vi "Pre Launch Init.vi"(11 "LoggingActor in":refnum<class "LoggingActor.lvclass">) -> (0 "error out":errorcluster, 3 "LoggingActor out":refnum<class "LoggingActor.lvclass">)   [LabVIEW 2022 SP3, in "LoggingActor.lvlib" / "LoggingActor.lvclass"]
doc: "(<B>Filename</B>: Actor Framework.lvlib:Actor.lvclass:Pre Launch Init.vi)\n\nDefines behavior that occurs after the Launch Actor method is invoked but before the actor's Actor Core method begins running.\n\nThe Pre Launch Init method is guaranteed to finish before the Launch Actor method returns to its caller and before the actor itself receives any messages. Any references that the Pre Launch Init method obtains are guaranteed to have the same lifetime as the actor itself. Any errors that the Pre Launch Init method returns will abort the launch.\n\nBy default, this method does nothing. A descendant class may override it to define behavior."
uses:
  LoggingActor.lvclass
  Logger/Source/Logger/_Level.ctl
  LoggingActor.lvclass/LoggingActor.ctl
  Logger/Source/FileHandler/FileHandler.lvclass
  C:/Users/jakub/repos/gh/sw4sys/lv-logging-actor/Logger/Source/Handler/Handler.lvclass
  <vilib>/ActorFramework/Actor/Actor.lvclass
  Logger/Source/Logger/Logger.lvclass
  DateTime/Source/DateTime.lvlib
  Logger/Source/Handler/Handler.lvclass
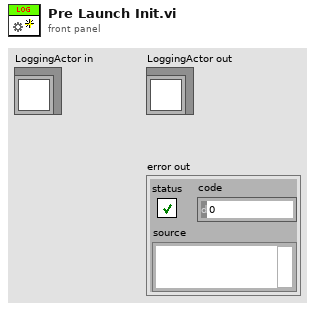
[diagram p1: front panel]
types:
  T1 = typedef "Logger.lvlib/Logger.lvclass/_Level.ctl" = enum16{"NOTSET", "DEBUG", "INFO", "WARNING", "ERROR", "CRITICAL"}
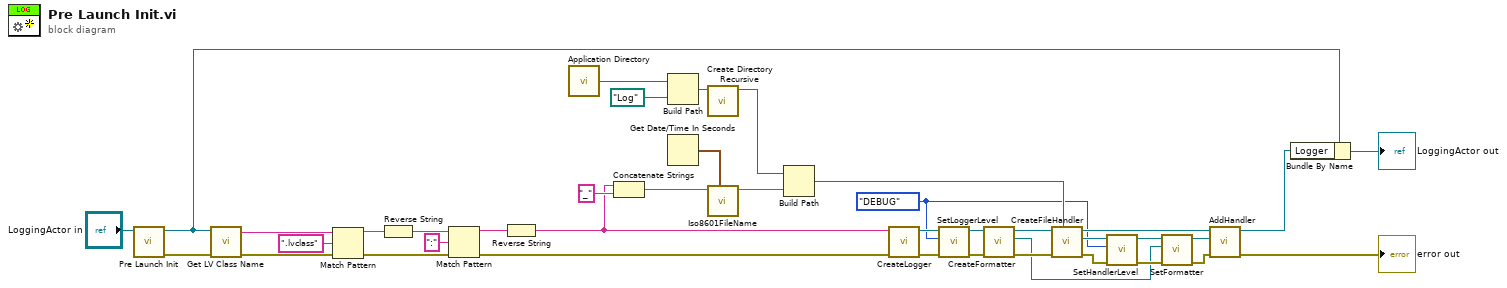
[diagram p0: block diagram]
diagram:
  w8 = _Level."DEBUG" ("Level")
  n1 = call-parent "Pre Launch Init.vi"("Actor in"="LoggingActor in") -> ("error out"=w36:errorcluster, "Actor out"=w10:refnum<class "LoggingActor.lvclass">)  [unwired: 9 in]
  n2 = call <vilib>:"Get LV Class Name.vi"("error in (no error)"=w36, "object"=w10) -> ("error out"=w35:errorcluster, "class name"=w4:string)  [unwired: 8 in]
  n3 = Match Pattern(string=w4, regular expression=".lvclass") -> (before substring=w6:string)  [unwired: 1 in, 3 out]
  n4 = Reverse String(1:w6) -> (0:w3:string)
  n5 = Match Pattern(string=w3, regular expression=":") -> (before substring=w2:string)  [unwired: 1 in, 3 out]
  n6 = Reverse String(1:w2) -> (0:w1:string)
  n7 = call <vilib>:"Application Directory.vi"() -> ("Application Directory"=w32:path)
  n8 = Concatenate Strings(w1, "_" ("Prefix ('')")) -> (w25:string)
  n9 = Build Path(base path=w32, name or relative path=path "Log") -> (appended path=w30:path)
  n10 = Get Date/Time In Seconds() -> (seconds since 1Jan1904=w28:timestamp)
  n11 = call <vilib>:"Create Directory Recursive.vi"("directory"=w30) -> ("directory copy"=w27:path)  [unwired: 4 in, 2 out]
  n12 = call "Iso8601FileName.vi"("TimeStamp"=w28, "Prefix ('')"=w25) -> ("FileName"=w29:string)  [unwired: 9 in]
  n13 = Build Path(base path=w27, name or relative path=w29) -> (appended path=w24:path)
  n14 = call "CreateLogger.vi"("error in (no error)"=w35, "Name"=w1) -> ("error out"=w37:errorcluster, "Logger"=w33:refnum<class "Logger.lvclass">)  [unwired: 8 in]
  n15 = call-dynamic "SetLoggerLevel.vi"("error in (no error)"=w37, "Level"=w8, "Logger in"=w33) -> ("error out"=w34:errorcluster, "Logger out"=w18:refnum<class "Logger.lvclass">)  [unwired: 7 in]
  n16 = call-dynamic "CreateFormatter.vi"("error in (no error)"=w34, "Logger in"=w18) -> ("error out"=w19:errorcluster, "Formatter"=w16:refnum<class "Formatter.lvclass">, "Logger out"=w17:refnum<class "Logger.lvclass">)  [unwired: 7 in]
  n17 = call-dynamic "CreateFileHandler.vi"("FIlePath"=w24, "error in (no error)"=w19, "Logger in"=w17) -> ("error out"=w21:errorcluster, "FileHandler"=w23:refnum<class "FileHandler.lvclass">, "Logger out"=w15:refnum<class "Logger.lvclass">)  [unwired: 6 in]
  n18 = call "SetHandlerLevel.vi"("error in (no error)"=w21, "Level"=w8, "Handler in"=w23) -> ("error out"=w20:errorcluster, "Handler out"=w22:refnum<class "Handler.lvclass">)  [unwired: 7 in]
  n19 = call "SetFormatter.vi"("error in (no error)"=w20, "Formatter in"=w16, "Handler in"=w22) -> ("error out"=w12:errorcluster, "Handler out"=w13:refnum<class "Handler.lvclass">)  [unwired: 6 in, 1 out]
  n20 = call-dynamic "AddHandler.vi"("error in (no error)"=w12, "Handler in"=w13, "Logger in"=w15) -> ("error out"=→"error out":errorcluster, "Logger out"=w14:refnum<class "Logger.lvclass">)  [unwired: 6 in, 1 out]
  n21 = Bundle By Name(cluster=w10, "Logger"=w14) -> (→"LoggingActor out":refnum<class "LoggingActor.lvclass">)
